vi "Build Monitor Boundaries.vi"(6 "Starting Address Offset":u16 format="%04x", 7 "Virtual Memory Unit in":refnum<class "Virtual Memory Unit.lvclass">, 8 "error in (no error)":errorcluster, 11 "Bus Monitor in":refnum<class "Bus Monitor.lvclass">) -> (0 "error out":errorcluster, 3 "Bus Monitor out":refnum<class "Bus Monitor.lvclass">, 5 "Virtual Memory Unit out":refnum<class "Virtual Memory Unit.lvclass">)   [LabVIEW 2020, in "BCI-1553 API.lvlib" / "Bus Monitor.lvclass"]
doc: "Generates all the data boundaries for the command and data words transacted for each bus. There are four groups:\n\nGroup 1: Bus A Command Words\nGroup 2: Bus A Data Words\nGroup 3: Bus B Command Words\nGroup 4: Bus B Data Words"
uses:
  Bus Monitor.lvclass
  Dependencies/Virtual Memory Unit/Virtual Memory Unit.lvclass
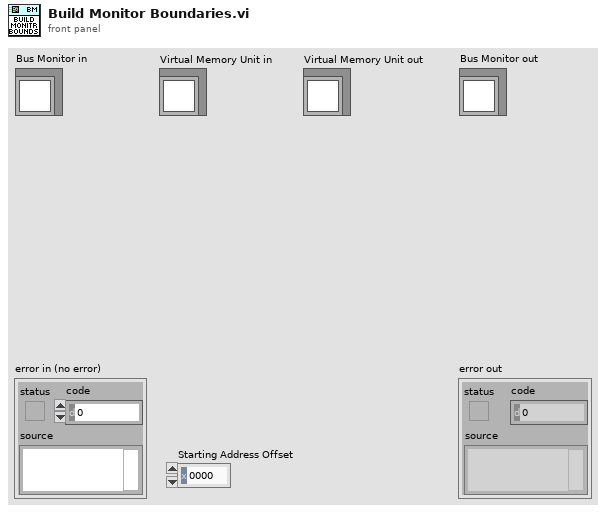
[diagram p1: front panel]
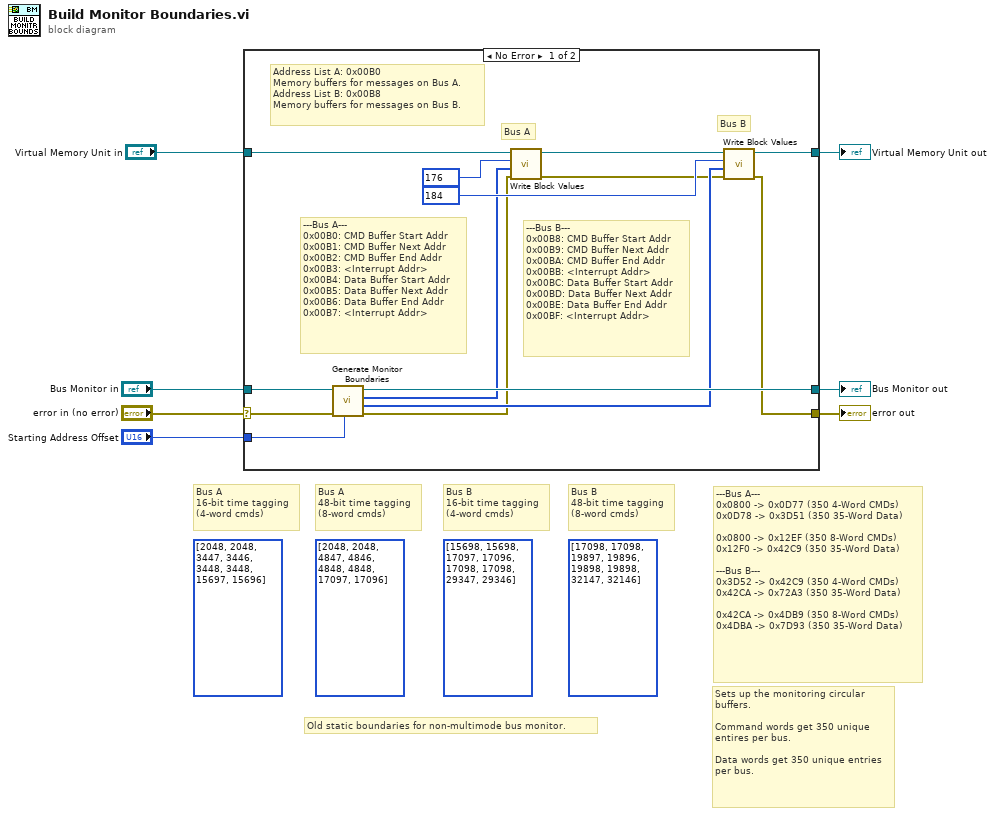
[diagram p0: block diagram]
diagram:
  (unwired) u16[] [15698, 15698, 17097, 17096, 17098, 17098, 29347, 29346]
  (unwired) u16[] [17098, 17098, 19897, 19896, 19898, 19898, 32147, 32146]
  (unwired) u16[] [2048, 2048, 4847, 4846, 4848, 4848, 17097, 17096]
  (unwired) u16[] [2048, 2048, 3447, 3446, 3448, 3448, 15697, 15696]
  # "Sets up the monitoring circular\nbuffers.\n\nCommand words get 350 unique\nentires per bus.\n\nData words get 350 unique entries\nper bus."
  # "---Bus A---\n0x0800 -> 0x0D77 (350 4-Word CMDs)\n0x0D78 -> 0x3D51 (350 35-Word Data)\n\n0x0800 -> 0x12EF (350 8-Word CMDs)\n0x12F0 -> 0x42C9 (350 35-Word Data)\n\n---Bus B---\n0x3D52 -> 0x42C9 (350 4-Word CMDs)\n0x42CA -> 0x72A3 (350 35-Word Data)\n\n0x42CA -> 0x4DB9 (350 8-Word CMDs)\n0x4DBA -> 0x7D93 (350 35-Word Data)"
  # "Old static boundaries for non-multimode bus monitor."
  # "Bus B\n16-bit time tagging\n(4-word cmds)"
  # "Bus B\n48-bit time tagging\n(8-word cmds)"
  # "Bus A\n16-bit time tagging\n(4-word cmds)"
  # "Bus A\n48-bit time tagging\n(8-word cmds)"
  n1 = case shown="No Error" "error in (no error)" {
    selector: "error in (no error)" -> [w15 w24]
    tunnel: [w8 w24] -> w6
    tunnel: [w13 w23] -> w4
    tunnel: "Bus Monitor in" -> [w16 w23]
    tunnel: "Virtual Memory Unit in" -> [w21 w22]
    tunnel: [w18 w22] -> w2
    tunnel: "Starting Address Offset" -> [w14 _]
    frame No Error {
      # "---Bus A---\n0x00B0: CMD Buffer Start Addr\n0x00B1: CMD Buffer Next Addr\n0x00B2: CMD Buffer End Addr\n0x00B3: <Interrupt Addr>\n0x00B4: Data Buffer Start Addr\n0x00B5: Data Buffer Next Addr\n0x00B6: Data Buffer End Addr\n0x00B7: <Interrupt Addr>"
      # "---Bus B---\n0x00B8: CMD Buffer Start Addr\n0x00B9: CMD Buffer Next Addr\n0x00BA: CMD Buffer End Addr\n0x00BB: <Interrupt Addr>\n0x00BC: Data Buffer Start Addr\n0x00BD: Data Buffer Next Addr\n0x00BE: Data Buffer End Addr\n0x00BF: <Interrupt Addr>"
      # "Bus B"
      # "Bus A"
      # "Address List A: 0x00B0\nMemory buffers for messages on Bus A.\nAddress List B: 0x00B8\nMemory buffers for messages on Bus B."
      n2 = call "Generate Monitor Boundaries.vi"("Starting Address Offset"=w14, "error in (no error)"=w15, "Bus Monitor in"=w16) -> ("error out"=w9:errorcluster, "Bus B Bounds"=w12:u16[], "Bus A Bounds"=w11:u16[], "Bus Monitor out"=w13:refnum<class "Bus Monitor.lvclass">)  [unwired: 5 in]
      n3 = call "Write Block Values.vi"("error in (no error)"=w9, "Write Block"=w11, "Start Index"=176, "Virtual Memory Unit in"=w21) -> ("error out"=w10:errorcluster, "Virtual Memory Unit out"=w19:refnum<class "Virtual Memory Unit.lvclass">)  [unwired: 6 in]
      n4 = call "Write Block Values.vi"("error in (no error)"=w10, "Write Block"=w12, "Start Index"=184, "Virtual Memory Unit in"=w19) -> ("error out"=w8:errorcluster, "Virtual Memory Unit out"=w18:refnum<class "Virtual Memory Unit.lvclass">)  [unwired: 6 in]
    }
    frame Error {
    }
  }
  "error out" <- w6
  "Bus Monitor out" <- w4
  "Virtual Memory Unit out" <- w2
